vi "ask_your_data.vi"(8 "error in (no error)":errorcluster, 10 "message_text":refnum<class "message_text.lvclass">, 11 "agent_simple_qa in":refnum<class "agent_simple_qa.lvclass">) -> (0 "error out":errorcluster, 2 "message_text_response":refnum<class "message_text.lvclass">, 3 "agent_simple_qa out":refnum<class "agent_simple_qa.lvclass">)   [LabVIEW 2020, in "agent_simple_qa.lvclass"]
uses:
  agent_simple_qa.lvclass
  models/message_text/message_text.lvclass
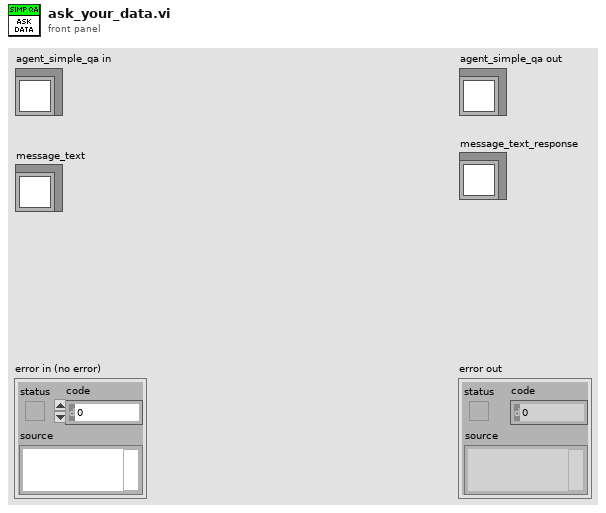
[diagram p1: front panel]
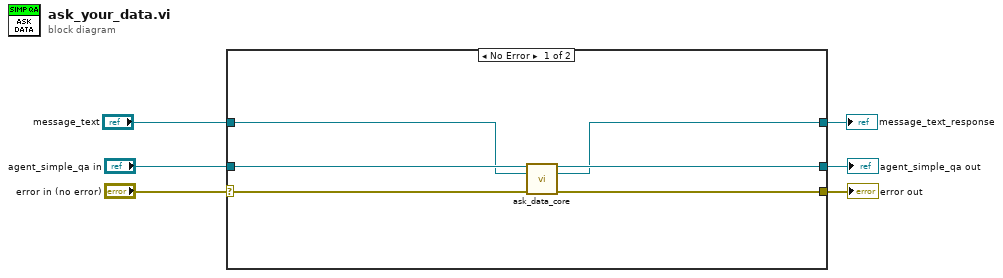
[diagram p0: block diagram]
diagram:
  n1 = case shown="No Error" "error in (no error)" {
    selector: "error in (no error)" -> [w10 w15]
    tunnel: [w9 w15] -> w5
    tunnel: [w11 w14] -> w3
    tunnel: "agent_simple_qa in" -> [w12 w14]
    tunnel: "message_text" -> [w8 w13]
    tunnel: [w7 w13] -> w1
    frame No Error {
      n2 = call-dynamic "ask_data_core.vi"("agent_simple_qa in"=w12, "message_text"=w8, "error in (no error)"=w10) -> ("agent_simple_qa out"=w11:refnum<class "agent_simple_qa.lvclass">, "message_text_response"=w7:refnum<class "message_text.lvclass">, "error out"=w9:errorcluster)  [unwired: 10 in]
    }
    frame Error {
    }
  }
  "error out" <- w5
  "agent_simple_qa out" <- w3
  "message_text_response" <- w1
